vi "Rx Data Available.vi"(8 "error in (no error)":errorcluster, 9 "Rx SubAddress (1-30)":u16, 10 "RT1?":bool, 11 "1553 Component in":refnum<class "1553 Component.lvclass">) -> (0 "error out":errorcluster, 2 "New Data Available?":bool, 3 "1553 Component out":refnum<class "1553 Component.lvclass">)   [LabVIEW 2020, in "BCI-1553 API.lvlib" / "1553 Component.lvclass"]
doc: "Attempts to check if the designated receive subaddress has received new data from a bus controller. If the subcomponent is not an RT, the method will return an error. The result of this method will latch high until the flag has been commanded to clear."
uses:
  1553 Component.lvclass
  1553 Component.lvclass/1553 Component.ctl
  Remote Terminal/Remote Terminal.lvclass
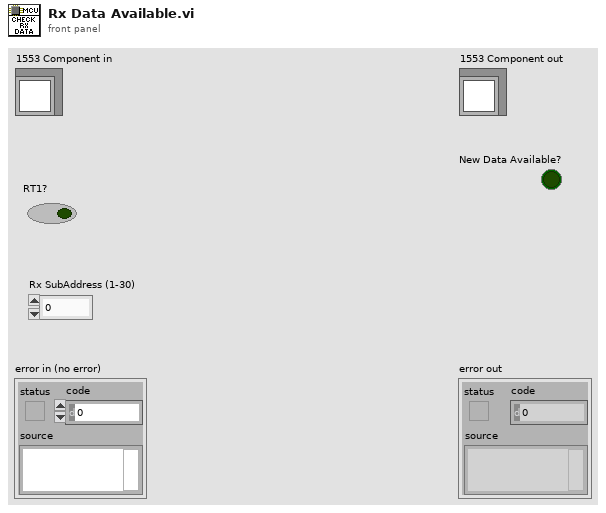
[diagram p1: front panel]
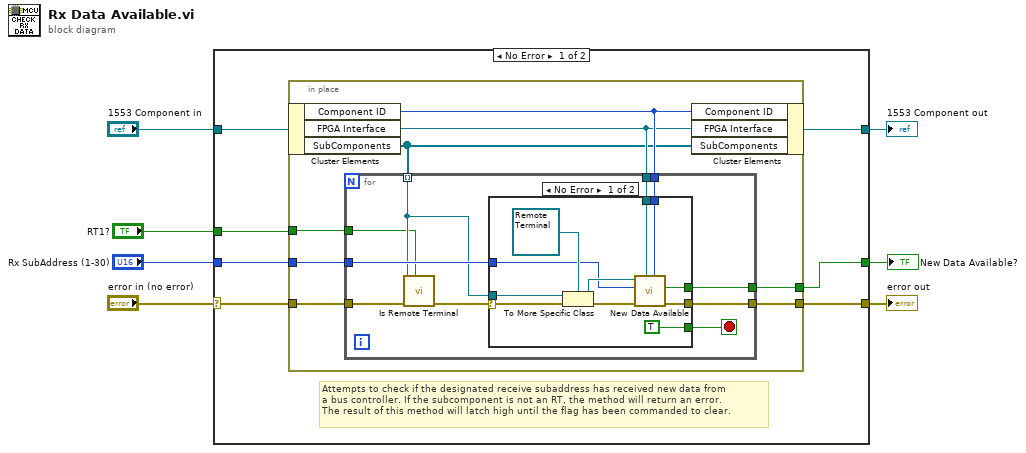
[diagram p0: block diagram]
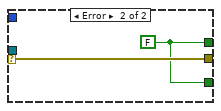
[diagram p2: hidden frame]
diagram:
  n1 = case shown="No Error" "error in (no error)" {
    selector: "error in (no error)" -> [w11 w47]
    tunnel: [w10 w47] -> w6
    tunnel: [w13 w46] -> w4
    tunnel: "1553 Component in" -> [w14 w46]
    tunnel: "Rx SubAddress (1-30)" -> [w12 _]
    tunnel: "RT1?" -> [w9 _]
    tunnel: [w8 _] -> w1
    frame No Error {
      # "Attempts to check if the designated receive subaddress has received new data from\na bus controller. If the subcomponent is not an RT, the method will return an error.\nThe result of this method will latch high until the flag has been commanded to clear."
      n2 = in-place {
        in-place-border: w11 -> [w19]
        in-place-border: [w20] -> w10
        in-place-border: w9 -> [w15]
        in-place-border: w12 -> [w18]
        in-place-border: [w17] -> w8
        n3 = in-place-cluster #1(w14) -> ("Component ID"=w22:u8, "FPGA Interface"=w21:refnum<class "FPGA Interface.lvclass">, "SubComponents"=w16:refnum<class "1553 SubComponent.lvclass">[])
        n4 = for {
          tunnel: w22 -> [w32]
          tunnel: w21 -> [w31]
          tunnel: w18 -> [w27]
          tunnel: [w26] -> w17
          tunnel: w16 -> [w25] mode=indexing
          tunnel: w15 -> [w24]
          tunnel: w19 -> [w29]
          tunnel: [w30] -> w20
          stop <- w23 stop-if-true
          n5 = call "Is Remote Terminal.vi"("RT1?"=w24, "error in (no error)"=w29, "1553 SubComponent"=w25) -> ("error out"=w28:errorcluster)  [unwired: 8 in]
          n6 = case shown="No Error" w28 {
            selector: w28 -> [w42 w45]
            tunnel: w32 -> [w36 _]
            tunnel: w31 -> [w37 _]
            tunnel: [w35 w45] -> w30
            tunnel: w25 -> [w43 _]
            tunnel: w27 -> [w39 _]
            tunnel: [w34 w44] -> w26
            tunnel: [TRUE w44] -> w23
            frame No Error {
              n7 = To More Specific Class(target class=refnum<class "Remote Terminal.lvclass"> refnum ("SLSC 1553 API.lvlib:Remote Terminal.lvclass"), reference=w43, error in=w42) -> (specific class reference=w41:refnum<class "Remote Terminal.lvclass">, error out=w38:errorcluster)
              n8 = call-dynamic "New Data Available.vi"("Component ID"=w36, "FPGA Interface"=w37, "error in (no error)"=w38, "Rx SubAddress (1-30)"=w39, "Remote Terminal in"=w41) -> ("error out"=w35:errorcluster, "New Data Available?"=w34:bool)  [unwired: 5 in]
            }
            frame Error {
              w44 = FALSE ("New Data Available?")
            }
          }
        }
        n9 = in-place-cluster #1("Component ID"=w22, "FPGA Interface"=w21, "SubComponents"=w16) -> (w13:refnum<class "1553 Component.lvclass">)
      }
    }
    frame Error {
    }
  }
  "error out" <- w6
  "1553 Component out" <- w4
  "New Data Available?" <- w1
